vi "TDMS文件配置.vi"(6 "时间间隔（s）":dbl, 8 "错误输入（无错误）":errorcluster, 9 "通道列表":string[](array[string]), 10 "时间标识输入控件":timestamp format="%<%x %.3X>T", 11 "文件路径":path) -> (0 "error out":errorcluster, 1 "通道列表":string[](array[string]), 2 "group name out":string, 3 "tdms file out":refnum<k34>)   [LabVIEW 2021]
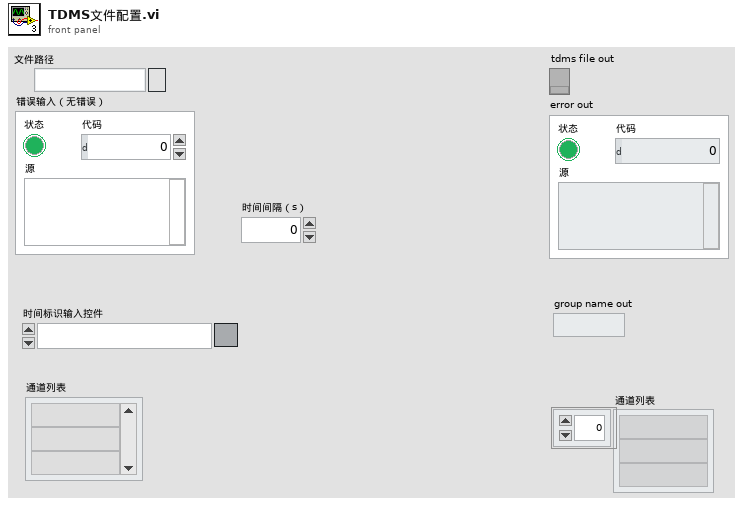
[diagram p1: front panel]
types:
  T1 = enum16{"open", "open or create", "create or replace", "create", "open (read-only)"}
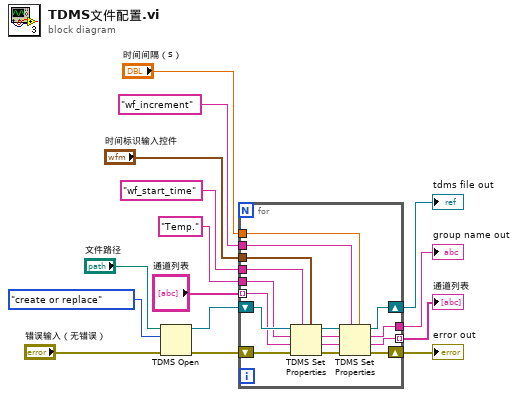
[diagram p0: block diagram]
diagram:
  n1 = TDMS Open(8:"错误输入（无错误）", 10:T1."create or replace" ("操作(0:open)"), 11:"文件路径") -> (0:w13:errorcluster, 3:w14:refnum<k34>)  [unwired: 4 in]
  n2 = for {
    tunnel: "wf_increment" -> [w22]
    tunnel: "Temp." ("组名称输入（无标题）") -> [w23]
    shift-right: [w26] -> w8
    shift-left: w14 -> [w31]
    shift-right: [w27] -> w7
    shift-left: w13 -> [w30]
    tunnel: "时间间隔（s）" -> [w21]
    tunnel: "通道列表" -> [w20] mode=indexing
    tunnel: "wf_start_time" -> [w19]
    tunnel: "时间标识输入控件" -> [w18]
    tunnel: [w17] -> w2
    tunnel: [w16] -> w1 mode=indexing
    n3 = TDMS Set Properties(5:w18, 7:w19, 8:w30, 9:w20, 10:w23, 11:w31) -> (0:w28:errorcluster, 1:w24:string, 2:w25:string, 3:w29:refnum<k34>)
    n4 = TDMS Set Properties(5:w21, 7:w22, 8:w28, 9:w24, 10:w25, 11:w29) -> (0:w27:errorcluster, 1:w16:string, 2:w17:string, 3:w26:refnum<k34>)
  }
  "tdms file out" <- w8
  "error out" <- w7
  "group name out" <- w2
  "通道列表" <- w1
